vi "Monitor Stream.vi"   [LabVIEW 2015, in "niInstr Streaming v1 FPGA.lvlib"]
doc: "This polymorphic VI provides several monitoring functions for FPGA streams. See the specific instances for details."
uses:
  <instrlib>/_niInstr/Streaming/v1/FPGA/niInstr Streaming v1 FPGA.lvlib
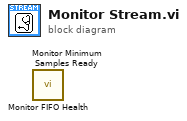
[diagram p0: block diagram]
diagram:
  n1 = call <instrlib>:"Monitor FIFO Health.vi"() -> ()  [unwired: 9 in, 3 out]
  n2 = call <instrlib>:"Monitor Minimum Samples Ready.vi"() -> ()  [unwired: 11 in, 1 out]
